vi "scale UI.vi"() -> ()   [LabVIEW 2013, in "Polynomial Scale editor node.lvclass"]
uses:
  Polynomial Scale editor node.lvclass
  <vilib>/NI/Configuration Framework/Node/NodeRef.ctl
  <vilib>/NI/Configuration Framework/Node/NISE_CEF_Node.lvclass
  <vilib>/NI/AMC/Message Queue.ctl
  <vilib>/NI/AMC/Message.ctl
  <vilib>/NI/Tools/Keyed Array/KeyedArray.ctl
  <vilib>/NI/Configuration Framework/Node/UserEventRef.ctl
  <vilib>/NI/Configuration Framework/Controls/EventCluster.ctl
  <vilib>/NI/Configuration Framework/Node/StopEvent.ctl
  <vilib>/NI/Configuration Framework/Node/RefreshUIEvent.ctl
  <vilib>/NI/Configuration Framework/Node/CacheState.ctl
  <vilib>/NI/Configuration Framework/Node/NodeChangeEvent.ctl
  <vilib>/NI/DCAF Table API/Table Manager/references.ctl
  <vilib>/NI/DCAF/Tag Editor Core/control module/editor node/channel action event.ctl
  <vilib>/NI/DCAF/Tag Editor Core/control module/editor node/dialog output action.ctl
  <vilib>/NI/Tag Bus Module Framework/channel/TBM channel.lvclass
  <vilib>/NI/Tag Bus/tag/tag descriptor.lvclass
  <vilib>/NI/DCAF/Tag Editor Core/Configuration Editor/Classes/Module editor node/module editor node.lvclass
  <vilib>/NI/DCAF Table API/Table Manager/object ref.ctl
  <vilib>/NI/DCAF/Tag Editor Core/Configuration Editor/Classes/Engine Parent/Engine Parent Editor Node.lvclass
  <vilib>/NI/DCAF Templates/DCAF Scaling/editor node/Scaling editor node.lvclass
  <vilib>/NI/Configuration Framework/NISE_CEF_TreeControl.lvlib
  <vilib>/NI/Tools/Keyed Array/Tools_KeyedArray.lvlib
  <vilib>/NI/AMC/AMC.lvlib
  <vilib>/NI/DCAF/Tag Editor Core/control module/editor node/control module editor.lvclass
  <vilib>/NI/DCAF Table API/Table Manager/Table Manager.lvclass
panel:
  out "Equation":string
  in  "Coefficients":dbl[](array[numeric])
  in  "node change":T1
  in  "cache state":T2
  in  "refresh UI":T3
  in  "stop event":T4
  in  "user event":T5
  in  "main queue":T6
  in  "node ref":T7
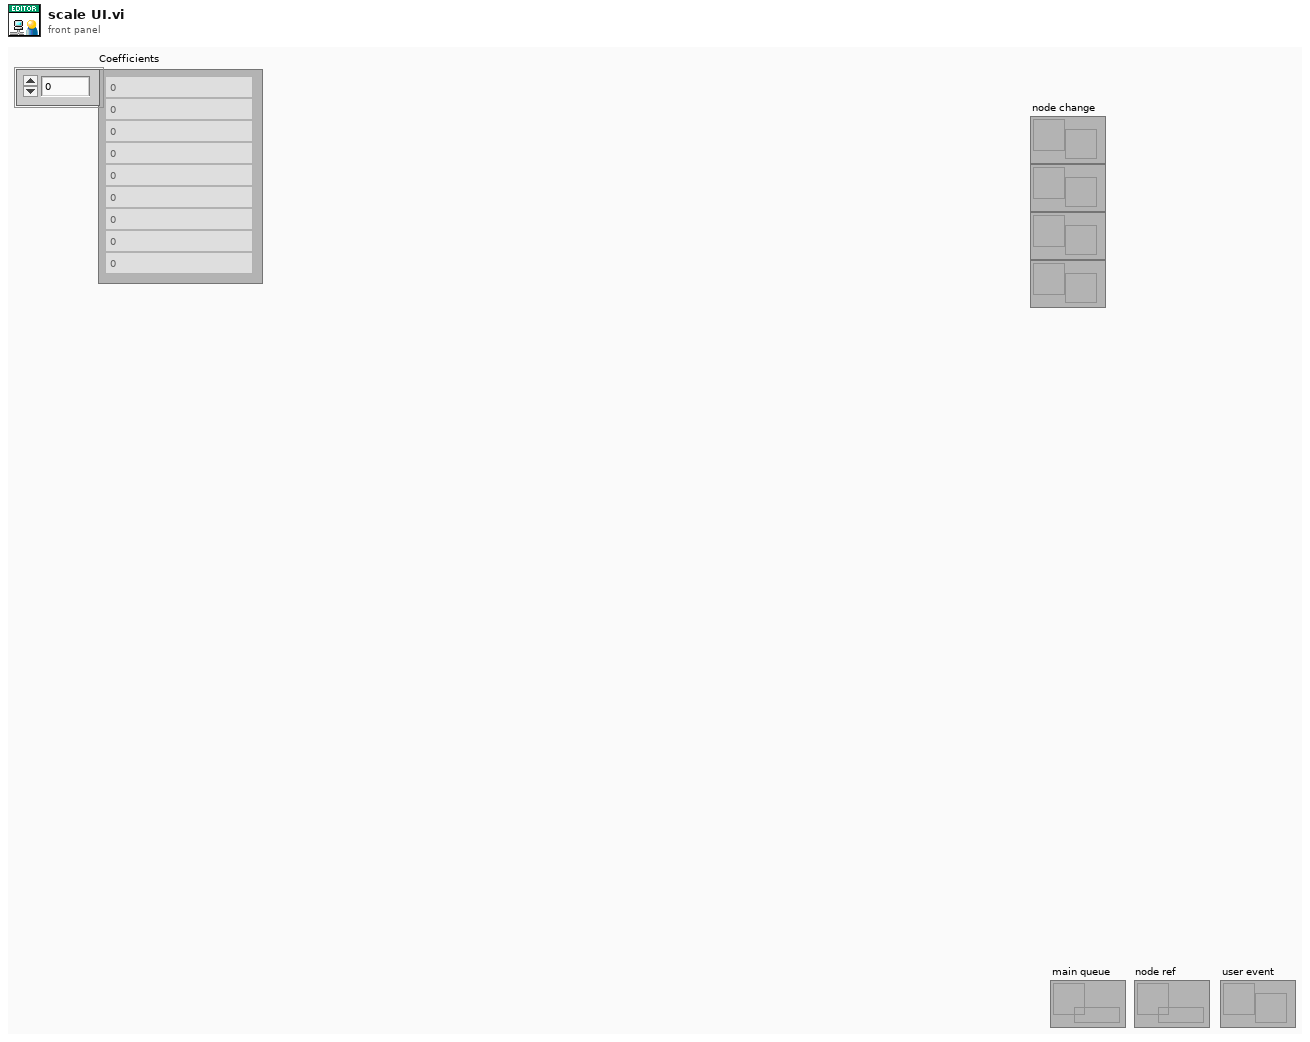
[diagram p1: front panel]
types:
  T1 = typedef "NISE_CEF_Node.lvclass/NodeChangeEvent.ctl" = refnum<user-event>
  T2 = typedef "NISE_CEF_Node.lvclass/CacheState.ctl" = refnum<user-event>
  T3 = typedef "NISE_CEF_Node.lvclass/RefreshUIEvent.ctl" = refnum<user-event>
  T4 = typedef "NISE_CEF_Node.lvclass/StopEvent.ctl" = refnum<user-event>
  T5 = typedef "NISE_CEF_Node.lvclass/UserEventRef.ctl" = refnum<user-event>
  T6 = typedef "AMC.lvlib/Message Queue.ctl" = refnum<queue>
  T7 = typedef "NISE_CEF_Node.lvclass/NodeRef.ctl" = refnum<data-value>
  T8 = typedef "Table Manager.lvlib/Table Manager.lvclass/object ref.ctl" = cluster{"engine":refnum<data-value>, "Node Ref":refnum<data-value>}
  T9 = typedef "Table Manager.lvlib/Table Manager.lvclass/references.ctl" = cluster{"stop event":T4, "refresh UI":T3, "cache state":T2, "node change":T1, "user event out":refnum<user-event>, "main queue":T6, "user event":T5}
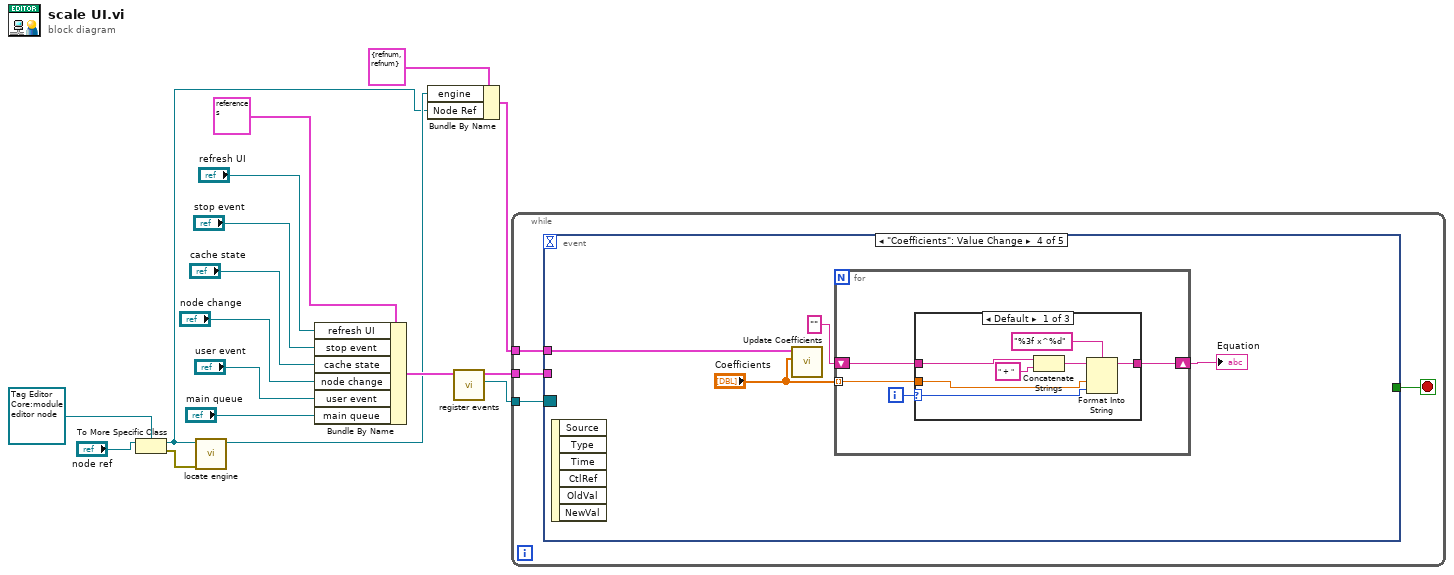
[diagram p0: block diagram]
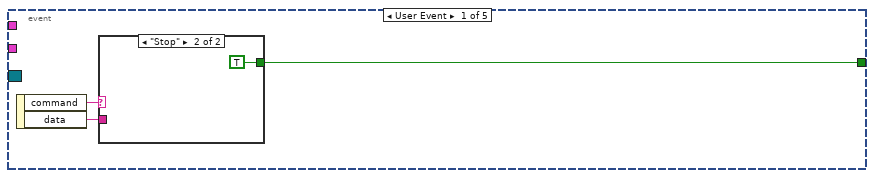
[diagram p2: hidden frame]
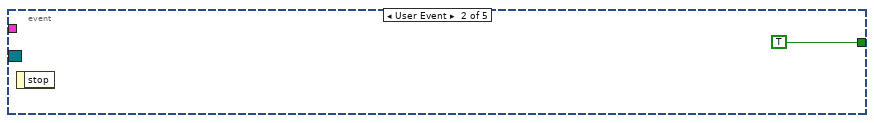
[diagram p4: hidden frame]
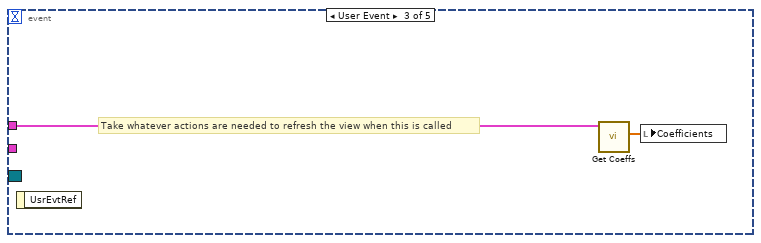
[diagram p5: hidden frame]
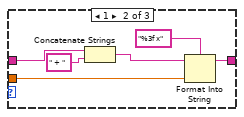
[diagram p6: hidden frame]
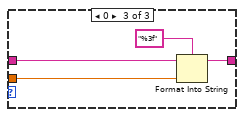
[diagram p7: hidden frame]
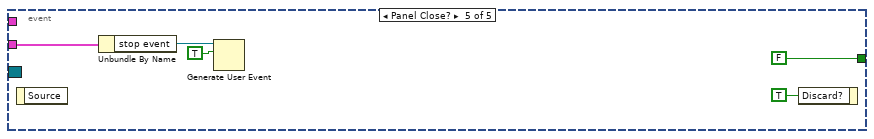
[diagram p8: hidden frame]
diagram:
  n1 = To More Specific Class(target class=refnum<data-value> refnum ("data value reference"), reference="node ref") -> (specific class reference=w2:refnum<data-value>, error out=w3:errorcluster)  [unwired: 1 in]
  n2 = call <vilib>:"locate engine.vi"("error in"=w3, "component"=w2) -> ("engine"=w5:refnum<data-value>)  [unwired: 8 in, 1 out]
  n3 = Bundle By Name(cluster=T9 {"stop event"=refnum, "refresh UI"=refnum, "cache state"=refnum, "node change"=refnum, "user event out"=refnum, "main queue"=refnum, "user event"=refnum} ("References in"), "refresh UI"="refresh UI", "stop event"="stop event", "cache state"="cache state", "node change"="node change", "user event"="user event", "main queue"="main queue") -> (w16:T9)
  n4 = Bundle By Name(cluster=T8 {"engine"=refnum, "Node Ref"=refnum} ("object refs"), "engine"=w5, "Node Ref"=w2) -> (w1:T8)
  n5 = call <vilib>:"register events.vi"("References"=w16) -> ("Event Registration Refnum"=w8:refnum<event-registration>, "References out"=w9:T9)  [unwired: 8 in, 1 out]
  n6 = while {
    tunnel: w9 -> [w21]
    tunnel: w8 -> [w20]
    tunnel: w1 -> [w18]
    stop <- w19 stop-if-true
    n7 = event shown="[3] \"Coefficients\": Value Change" {
      selector: w20 -> [_ _ _ _ _]
      dyn-events: _ -> [_ _ _ _ _]
      timeout: _ -> [_ _ _ _ _]
      tunnel: [w24 TRUE _ _ FALSE] -> w19
      tunnel: w21 -> [_ _ _ _ w55]
      tunnel: w18 -> [_ _ w28 w32 _]
      event User Event {
        n8 = event-data() -> ("command"=w23:string, "data"=w22:string)  [unwired: 1 in]
        n9 = case shown="\"Stop\"" w23 {
          tunnel: [_ TRUE] -> w24
          tunnel: w22 -> [_ _]
          frame Default {
          }
          frame "Stop" {
          }
        }
      }
      event User Event {
        n10 = event-data() -> ()  [unwired: 1 in, 1 out]
      }
      event User Event {
        # "Take whatever actions are needed to refresh the view when this is called"
        n11 = event-data() -> ()  [unwired: 1 in, 1 out]
        n12 = call "Get Coeffs.vi"("references"=w28) -> ("Coefficients"=w27:dbl[])  [unwired: 8 in, 2 out]
        n13 = local write "Coefficients"(w27) -> ()
      }
      event "Coefficients": Value Change {
        n14 = event-data() -> ()  [unwired: 1 in, 6 out]
        n15 = call "Update Coefficients.vi"("coeffs"="Coefficients", "references"=w32) -> ()  [unwired: 9 in, 1 out]
        n16 = for {
          tunnel: "Coefficients" -> [w34] mode=indexing
          shift-right: [w33] -> w29
          shift-left: "" ("format string") -> [w35]
          i -> [w36]
          n17 = case shown="Default" w36 {
            selector: w36 -> [w39 _ _]
            tunnel: w35 -> [w42 w48 w53]
            tunnel: w34 -> [w38 w45 w51]
            tunnel: [w37 w44 w50] -> w33
            frame Default {
              n18 = Concatenate Strings(w42, " + " ("string")) -> (w41:string)
              n19 = Format Into String(format string="%3f x^%d", initial string=w41, w38, w39) -> (resulting string=w37:string)  [unwired: 1 in, 1 out]
            }
            frame 1 {
              n20 = Concatenate Strings(w48, " + " ("string")) -> (w47:string)
              n21 = Format Into String(format string="%3f x", initial string=w47, w45) -> (resulting string=w44:string)  [unwired: 1 in, 1 out]
            }
            frame 0 {
              n22 = Format Into String(format string="%3f", initial string=w53, w51) -> (resulting string=w50:string)  [unwired: 1 in, 1 out]
            }
          }
        }
        "Equation" <- w29
      }
      event Panel Close? {
        n23 = event-data() -> ()  [unwired: 1 in, 1 out]
        n24 = Unbundle By Name(w55) -> ("stop event"=w54:T4)
        n25 = Generate User Event(user event=w54, event data cluster=TRUE ("event data")) -> ()  [unwired: 2 in, 2 out]
        n26 = event-data("Discard?"=TRUE) -> ()  [unwired: 1 in, 1 out]
      }
    }
  }
